vi "joystick_rio.vi"() -> ()   [LabVIEW 2017]
uses:
  <vilib>/myRIO/Express VI/Onboard IO/PWM/PWM Express VI.xnode
  <vilib>/myRIO/Instrument Drivers/Onboard IO/PWM/vis/Set Duty Cycle and Frequency.vi
  <vilib>/myRIO/Instrument Drivers/Onboard IO/PWM/PWM.lvlib
  <vilib>/myRIO/Instrument Drivers/Onboard IO/PWM/typedefs/PWM Configuration.ctl
  <vilib>/myRIO/Common/Instrument Driver Framework/myRIO v1.0/PWM/typedefs/PWM Channels Enum.ctl
  <vilib>/myRIO/Common/Instrument Driver Framework/Utilities/typedefs/Generic FPGA Reference.ctl
  <vilib>/myRIO/Common/Instrument Driver Framework/Utilities/typedefs/myRIO v1.0 Reference.ctl
  <vilib>/myRIO/Common/Instrument Driver Framework/Utilities/typedefs/Hardware Version Enum.ctl
  <vilib>/myRIO/Common/Instrument Driver Framework/Utilities/typedefs/myRIO Generic Hardware Reference.ctl
  <vilib>/myRIO/Instrument Drivers/Onboard IO/PWM/typedefs/PWM Reference.ctl
  <vilib>/myRIO/Instrument Drivers/Onboard IO/PWM/vis/myRIO PWM Open.xnode
  <vilib>/myRIO/Common/Instrument Driver Framework/Utilities/vis/Is FPGA Ref Available.vi
  <vilib>/myRIO/Common/Instrument Driver Framework/myRIO v1.0/PWM/vis/myRIO v1.1 Open PWM.vi
  <vilib>/userdefined/High Color/nirio_resource_hc.ctl
  <vilib>/myRIO/Express VI/Onboard Devices/LED/LED Express VI.xnode
  <vilib>/myRIO/Instrument Drivers/Onboard IO/DIO/vis/Write.vi
  <vilib>/myRIO/Instrument Drivers/Onboard IO/DIO/DIO.lvlib
  <vilib>/myRIO/Common/Instrument Driver Framework/myRIO v1.0/DIO/typedefs/DIO Channels Enum.ctl
  <vilib>/myRIO/Common/Instrument Driver Framework/myRIO v1.0/DIO/typedefs/DIO Channels List.ctl
  <vilib>/myRIO/Instrument Drivers/Onboard IO/DIO/typedefs/DIO Reference.ctl
  <vilib>/myRIO/Instrument Drivers/Onboard IO/DIO/vis/myRIO DIO Open.xnode
  <vilib>/myRIO/Common/Instrument Driver Framework/myRIO v1.0/DIO/vis/myRIO v1.1 Open DIO.vi
panel:
  out "Variable3":i32
  out "Variable2":i32
  in  "stop":bool
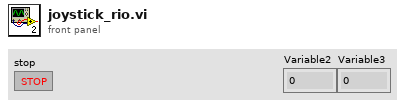
[diagram p1: front panel]
types:
  T1 = typedef "DIO.lvlib/DIO Reference.ctl" = cluster{"myRIO Reference":T2, "DIO Channels List":T6}
  T2 = typedef "myRIO Generic Hardware Reference.ctl" = cluster{"myRIO Model":T3, "myRIO Hardware Reference":T4}
  T3 = typedef "Hardware Version Enum.ctl" = enum16{"Unknown", "myRIO-1900", "myRIO-1950", "roboRIO", "NI ELVIS RIO CM"}
  T4 = typedef "myRIO v1.0 Reference.ctl" = cluster{"Generic FPGA Reference":T5, "Allow multiple opens":bool}
  T5 = typedef "Generic FPGA Reference.ctl" = refnum<k20>
  T6 = typedef "DIO Channels List.ctl" = T7[]
  T7 = typedef "DIO Channels Enum.ctl" = enum16{"Not Connected", "C/DIO0", "C/DIO1", "C/DIO2", "C/DIO3", "C/DIO4", "C/DIO5", "C/DIO6", "C/DIO7", "A/DIO0", "A/DIO1", "A/DIO2", "A/DIO3", "A/DIO4", "A/DIO5", "A/DIO6", "A/DIO7", "A/DIO8", "A/DIO9", "A/DIO10", "A/DIO11", "A/DIO12", "A/DIO13", "A/DIO14", "A/DIO15", "B/DIO0", "B/DIO1", "B/DIO2", "B/DIO3", "B/DIO4", "B/DIO5", "B/DIO6", "B/DIO7", "B/DIO8", "B/DIO9", "B/DIO10", "B/DIO11", "B/DIO12", "B/DIO13", "B/DIO14", "B/DIO15", "LED0", "LED1", "LED2", "LED3", "Button0", "DIO/DIO0", "DIO/DIO1", "DIO/DIO2", "DIO/DIO3", "DIO/DIO4", "DIO/DIO5", "DIO/DIO6", "DIO/DIO7", "DIO/DIO8", "DIO/DIO9", "SPI/CS0", "SPI/CS1", "SPI/CS2", "SPI/CS3", "LED RADIO (Green)", "LED RADIO (Red)", "LED COMM (Green)", "LED COMM (Red)", "LED MODE (Green)", "LED MODE (Red)"}
  T8 = typedef "nirio_resource_hc.ctl" = tag
  T9 = typedef "PWM.lvlib/PWM Reference.ctl" = cluster{"myRIO Reference":T2, "PWM Channels Enum":T10, "PWM Configuration":T11}
  T10 = typedef "PWM Channels Enum.ctl" = enum16{"Not Connected", "C/PWM0", "C/PWM1", "A/PWM0", "A/PWM1", "A/PWM2", "B/PWM0", "B/PWM1", "B/PWM2", "PWM/PWM0", "PWM/PWM1", "PWM/PWM2", "PWM/PWM3", "PWM/PWM4", "PWM/PWM5", "PWM/PWM6", "PWM/PWM7", "PWM/PWM8", "PWM/PWM9"}
  T11 = typedef "PWM.lvlib/PWM Configuration.ctl" = cluster{"Frequency":dbl, "Duty Cycle":dbl}
  T12 = cluster{"Array of Boolean[0]":bool, "Array of Boolean[1]":bool, "Array of Boolean[2]":bool, "Array of Boolean[3]":bool, "Array of Boolean[4]":bool, "Array of Boolean[5]":bool, "Array of Boolean[6]":bool, "Array of Boolean[7]":bool, "Array of Boolean[8]":bool}
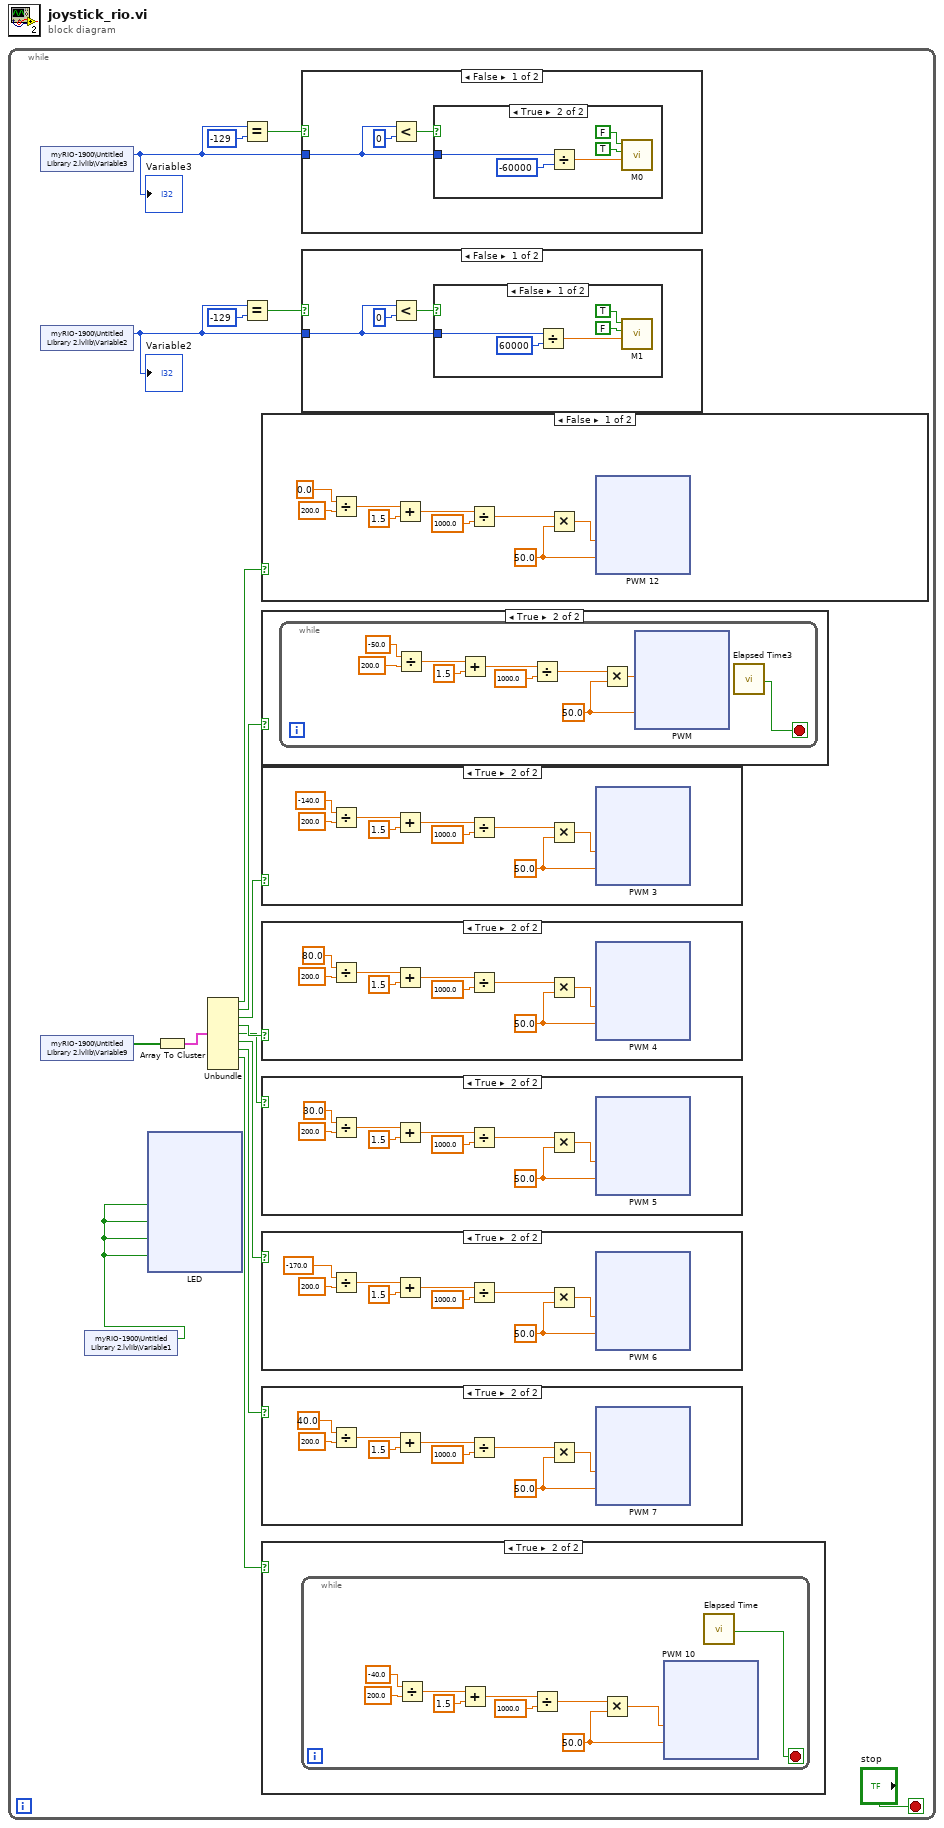
[diagram p0: block diagram]
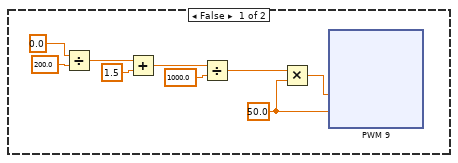
[diagram p2: hidden frame]
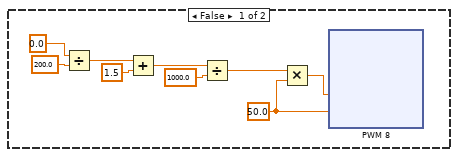
[diagram p3: hidden frame]
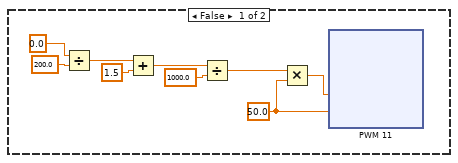
[diagram p8: hidden frame]
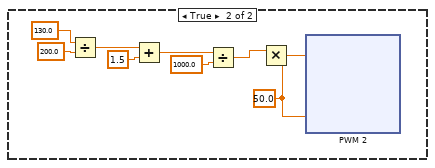
[diagram p9: hidden frame]
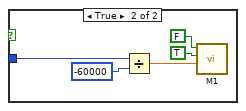
[diagram p10: hidden frame]
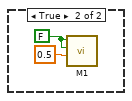
[diagram p11: hidden frame]
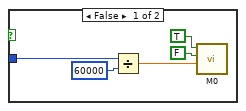
[diagram p12: hidden frame]
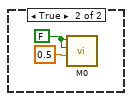
[diagram p13: hidden frame]
diagram:
  n1 = while {
    stop <- "stop" stop-if-true
    n2 = shared-variable "myRIO-1900\\Untitled Library 2.lvlib\\Variable3"() -> (w14:i32)  [unwired: 1 in, 1 out]
    "Variable3" <- w14
    n3 = shared-variable "myRIO-1900\\Untitled Library 2.lvlib\\Variable2"() -> (w15:i32)  [unwired: 1 in, 1 out]
    "Variable2" <- w15
    n4 = shared-variable "myRIO-1900\\Untitled Library 2.lvlib\\Variable9"() -> (w13:bool[])  [unwired: 1 in, 1 out]
    n5 = shared-variable "myRIO-1900\\Untitled Library 2.lvlib\\Variable1"() -> (w1:bool)  [unwired: 1 in, 1 out]
    n6 = xnode "LED"("LED0"=w1, "LED1"=w1, "LED2"=w1, "LED3"=w1) -> ()  [unwired: 1 in, 1 out]
    n7 = Array To Cluster(array=w13) -> (cluster=w12:T12)
    n8 = Unbundle(w12) -> ("Array of Boolean[0]"=w11:bool, "Array of Boolean[1]"=w10:bool, "Array of Boolean[2]"=w9:bool, "Array of Boolean[3]"=w8:bool, "Array of Boolean[4]"=w7:bool, "Array of Boolean[5]"=w6:bool, "Array of Boolean[6]"=w3:bool, "Array of Boolean[7]"=w2:bool)  [unwired: 1 out]
    n9 = Equal?(x=w14, y=-129) -> (x = y?=w4:bool)
    n10 = Equal?(x=w15, y=-129) -> (x = y?=w5:bool)
    n11 = case shown="False" w11 {
      frame False {
        w503 = 50.0 ("Frequency [Hz]")
        n12 = Divide(x=0.0, y=200.0) -> (x/y=w505:dbl)
        n13 = Add(x=w505, y=1.5) -> (x+y=w506:dbl)
        n14 = Divide(x=w506, y=1000.0) -> (x/y=w507:dbl)
        n15 = Multiply(x=w507, y=w503) -> (x*y=w504:dbl)
        n16 = xnode "PWM 12"("Duty Cycle"=w504, "Frequency [Hz]"=w503) -> ()  [unwired: 1 in, 1 out]
      }
      frame True {
        w547 = 50.0 ("Frequency [Hz]")
        n17 = Divide(x=130.0, y=200.0) -> (x/y=w549:dbl)
        n18 = Add(x=w549, y=1.5) -> (x+y=w550:dbl)
        n19 = Divide(x=w550, y=1000.0) -> (x/y=w551:dbl)
        n20 = Multiply(x=w551, y=w547) -> (x*y=w548:dbl)
        n21 = xnode "PWM 2"("Duty Cycle"=w548, "Frequency [Hz]"=w547) -> ()  [unwired: 1 in, 1 out]
      }
    }
    n22 = case shown="True" w10 {
      frame False {
        w414 = 50.0 ("Frequency [Hz]")
        n23 = Divide(x=0.0, y=200.0) -> (x/y=w416:dbl)
        n24 = Add(x=w416, y=1.5) -> (x+y=w417:dbl)
        n25 = Divide(x=w417, y=1000.0) -> (x/y=w418:dbl)
        n26 = Multiply(x=w418, y=w414) -> (x*y=w415:dbl)
        n27 = xnode "PWM 11"("Duty Cycle"=w415, "Frequency [Hz]"=w414) -> ()  [unwired: 1 in, 1 out]
      }
      frame True {
        n28 = while {
          stop <- w454 stop-if-true
          w459 = 50.0 ("Frequency [Hz]")
          n29 = Divide(x=-50.0, y=200.0) -> (x/y=w461:dbl)
          n30 = Add(x=w461, y=1.5) -> (x+y=w462:dbl)
          n31 = Divide(x=w462, y=1000.0) -> (x/y=w463:dbl)
          n32 = Multiply(x=w463, y=w459) -> (x*y=w460:dbl)
          n33 = xnode "PWM"("Duty Cycle"=w460, "Frequency [Hz]"=w459) -> ()  [unwired: 1 in, 1 out]
          n34 = call "Elapsed Time3"() -> ("Time has Elapsed"=w454:bool)  [unwired: 12 in, 7 out]
        }
      }
    }
    n35 = case shown="True" w9 {
      frame False {
      }
      frame True {
        w370 = 50.0 ("Frequency [Hz]")
        n36 = Divide(x=-140.0, y=200.0) -> (x/y=w373:dbl)
        n37 = Add(x=w373, y=1.5) -> (x+y=w372:dbl)
        n38 = Divide(x=w372, y=1000.0) -> (x/y=w371:dbl)
        n39 = Multiply(x=w371, y=w370) -> (x*y=w374:dbl)
        n40 = xnode "PWM 3"("Duty Cycle"=w374, "Frequency [Hz]"=w370) -> ()  [unwired: 1 in, 1 out]
      }
    }
    n41 = case shown="True" w8 {
      frame False {
      }
      frame True {
        w326 = 50.0 ("Frequency [Hz]")
        n42 = Divide(x=80.0, y=200.0) -> (x/y=w328:dbl)
        n43 = Add(x=w328, y=1.5) -> (x+y=w329:dbl)
        n44 = Divide(x=w329, y=1000.0) -> (x/y=w330:dbl)
        n45 = Multiply(x=w330, y=w326) -> (x*y=w327:dbl)
        n46 = xnode "PWM 4"("Duty Cycle"=w327, "Frequency [Hz]"=w326) -> ()  [unwired: 1 in, 1 out]
      }
    }
    n47 = case shown="True" w7 {
      frame False {
      }
      frame True {
        w282 = 50.0 ("Frequency [Hz]")
        n48 = Divide(x=30.0, y=200.0) -> (x/y=w284:dbl)
        n49 = Add(x=w284, y=1.5) -> (x+y=w285:dbl)
        n50 = Divide(x=w285, y=1000.0) -> (x/y=w286:dbl)
        n51 = Multiply(x=w286, y=w282) -> (x*y=w283:dbl)
        n52 = xnode "PWM 5"("Duty Cycle"=w283, "Frequency [Hz]"=w282) -> ()  [unwired: 1 in, 1 out]
      }
    }
    n53 = case shown="True" w6 {
      frame False {
      }
      frame True {
        w238 = 50.0 ("Frequency [Hz]")
        n54 = Divide(x=-170.0, y=200.0) -> (x/y=w240:dbl)
        n55 = Add(x=w240, y=1.5) -> (x+y=w241:dbl)
        n56 = Divide(x=w241, y=1000.0) -> (x/y=w242:dbl)
        n57 = Multiply(x=w242, y=w238) -> (x*y=w239:dbl)
        n58 = xnode "PWM 6"("Duty Cycle"=w239, "Frequency [Hz]"=w238) -> ()  [unwired: 1 in, 1 out]
      }
    }
    n59 = case shown="True" w3 {
      frame False {
        w150 = 50.0 ("Frequency [Hz]")
        n60 = Divide(x=0.0, y=200.0) -> (x/y=w152:dbl)
        n61 = Add(x=w152, y=1.5) -> (x+y=w153:dbl)
        n62 = Divide(x=w153, y=1000.0) -> (x/y=w154:dbl)
        n63 = Multiply(x=w154, y=w150) -> (x*y=w151:dbl)
        n64 = xnode "PWM 8"("Duty Cycle"=w151, "Frequency [Hz]"=w150) -> ()  [unwired: 1 in, 1 out]
      }
      frame True {
        w194 = 50.0 ("Frequency [Hz]")
        n65 = Divide(x=40.0, y=200.0) -> (x/y=w196:dbl)
        n66 = Add(x=w196, y=1.5) -> (x+y=w197:dbl)
        n67 = Divide(x=w197, y=1000.0) -> (x/y=w198:dbl)
        n68 = Multiply(x=w198, y=w194) -> (x*y=w195:dbl)
        n69 = xnode "PWM 7"("Duty Cycle"=w195, "Frequency [Hz]"=w194) -> ()  [unwired: 1 in, 1 out]
      }
    }
    n70 = case shown="True" w2 {
      frame False {
        w61 = 50.0 ("Frequency [Hz]")
        n71 = Divide(x=0.0, y=200.0) -> (x/y=w63:dbl)
        n72 = Add(x=w63, y=1.5) -> (x+y=w64:dbl)
        n73 = Divide(x=w64, y=1000.0) -> (x/y=w65:dbl)
        n74 = Multiply(x=w65, y=w61) -> (x*y=w62:dbl)
        n75 = xnode "PWM 9"("Duty Cycle"=w62, "Frequency [Hz]"=w61) -> ()  [unwired: 1 in, 1 out]
      }
      frame True {
        n76 = while {
          stop <- w101 stop-if-true
          w106 = 50.0 ("Frequency [Hz]")
          n77 = Divide(x=-40.0, y=200.0) -> (x/y=w108:dbl)
          n78 = Add(x=w108, y=1.5) -> (x+y=w109:dbl)
          n79 = Divide(x=w109, y=1000.0) -> (x/y=w110:dbl)
          n80 = Multiply(x=w110, y=w106) -> (x*y=w107:dbl)
          n81 = xnode "PWM 10"("Duty Cycle"=w107, "Frequency [Hz]"=w106) -> ()  [unwired: 1 in, 1 out]
          n82 = call "Elapsed Time"() -> ("Time has Elapsed"=w101:bool)  [unwired: 12 in, 7 out]
        }
      }
    }
    n83 = case shown="False" w4 {
      tunnel: w14 -> [w602 _]
      frame False {
        n84 = Less?(x=w602, y=0) -> (x < y?=w603:bool)
        n85 = case shown="True" w603 {
          tunnel: w602 -> [w606 w612]
          frame False {
            n86 = Divide(x=w606, y=60000) -> (x/y=w605:dbl)
            n87 = call "M0.vi"("Duty Cycle"=w605, "назад"=FALSE ("вперед"), "вперед"=TRUE) -> ()  [unwired: 8 in, 1 out]
          }
          frame True {
            n88 = Divide(x=w612, y=-60000) -> (x/y=w610:dbl)
            n89 = call "M0.vi"("Duty Cycle"=w610, "назад"=TRUE ("вперед"), "вперед"=FALSE) -> ()  [unwired: 8 in, 1 out]
          }
        }
      }
      frame True {
        w616 = FALSE
        n90 = call "M0.vi"("Duty Cycle"=0.5, "назад"=w616, "вперед"=w616) -> ()  [unwired: 8 in, 1 out]
      }
    }
    n91 = case shown="False" w5 {
      tunnel: w15 -> [w587 _]
      frame False {
        n92 = Less?(x=w587, y=0) -> (x < y?=w588:bool)
        n93 = case shown="False" w588 {
          tunnel: w587 -> [w591 w595]
          frame False {
            n94 = Divide(x=w591, y=60000) -> (x/y=w590:dbl)
            n95 = call "M1.vi"("Duty Cycle"=w590, "назад"=FALSE, "вперед"=TRUE ("назад")) -> ()  [unwired: 8 in, 1 out]
          }
          frame True {
            n96 = Divide(x=w595, y=-60000) -> (x/y=w596:dbl)
            n97 = call "M1.vi"("Duty Cycle"=w596, "назад"=TRUE, "вперед"=FALSE ("назад")) -> ()  [unwired: 8 in, 1 out]
          }
        }
      }
      frame True {
        w601 = FALSE
        n98 = call "M1.vi"("Duty Cycle"=0.5, "назад"=w601, "вперед"=w601) -> ()  [unwired: 8 in, 1 out]
      }
    }
  }
